vi "手-自动.vi"() -> (3 "Start":bool)   [LabVIEW 2020]
uses:
  Libraries/S7/S7.lvlib
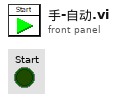
[diagram p1: front panel]
types:
  T1 = typedef "S7.lvlib/Read_Data (Reply Payload)--cluster.ctl" = cluster{"读取成功":bool, "数据":u32[], "Read_Data_error":errorcluster}
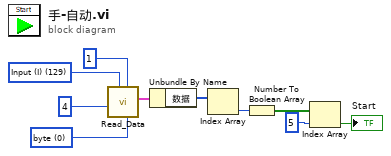
[diagram p0: block diagram]
diagram:
  w8 = u16 0 items=["byte", "word", "Dword"] ("数据类型")
  w9 = u8 129 items=["I/O (P)"=128, "Input (I)"=129, "Output (Q)"=130, "Bit Memory (M)"=131, "Data (DB)"=132, "Instance Data (DI)"=133, "Local Data (L)"=134, "Predecessor Local Data (VL)"=135] ("寄存器类型")
  n1 = call "Read_Data.vi"("数据类型"=w8, "读取长度"=u16 1, "寄存器类型"=w9, "起始地址"=u32 4) -> ("Reply Payload"=w6:T1)  [unwired: 5 in, 2 out]
  n2 = Unbundle By Name(w6) -> ("数据"=w5:u32[])
  n3 = Index Array(array=w5) -> (element=w4:u32)  [unwired: 1 in]
  n4 = Number To Boolean Array(number=w4) -> (Boolean array=w3:bool[])
  n5 = Index Array(array=w3, index=5 ("索引")) -> (element=→"Start":bool)
